vi "[RT] Finite Acq wSubset Reads.vi"() -> ()   [LabVIEW 2015]
doc: "A finite acquisition allocates exactly enough memory to hold all of the requested samples per channel. The rwfm_Read(poly).vi has a control named \"Samps Read per Chan\" that you can use to specify the block size returned by each Read call. In effect you can read a large finite acquisition in multiple small subsets."
uses:
  <vilib>/rvi/interface/nirviOpenFPGA/nirviOpenFPGA.xnode
  <vilib>/rvi/interface/nirviCloseFPGA/nirviCloseFPGA.xnode
  <vilib>/NI/cRIO Wfm/cRIO Wfm.lvlib
  <vilib>/NI/cRIO Wfm/AcqRead(Wfm).vi
  C/Program Files (x86)/National Instruments/LabVIEW 2015/ProjectTemplates/Source/cRIOWfm/FPGA Bitfiles/DeltaSigMain_9074.lvbitx
  C:/Program Files (x86)/National Instruments/LabVIEW 2015/ProjectTemplates/Source/cRIOWfm/FPGA/[FPGA] DeltaSig Main.vi
  C/Program Files (x86)/National Instruments/LabVIEW 2015/ProjectTemplates/Source/cRIOWfm/FPGA Bitfiles/SARAcqMain_9074.lvbitx
  C:/Program Files (x86)/National Instruments/LabVIEW 2015/ProjectTemplates/Source/cRIOWfm/FPGA/[FPGA] SAR Acq Main.vi
  <vilib>/NI/cRIO Wfm/DynamicFPGAref.ctl
  <vilib>/FPGAPlugInAG/Dynamic/niLvFpga_Close_Dynamic.vi
  <vilib>/NI/cRIO Wfm/ChannelConfig.ctl
panel:
  in  "Sample Rate":u32=51200
  in  "Channel Info":T1=[{"Channel Name"="Mod1/ai0", "Sensitivity mV_EU"=1000.0, "EU"="V", "dB Ref EU"=1.0}, {"Channel Name"="Mod1/ai1", "Sensitivity mV_EU"=1000.0, "EU"="V", "dB Ref EU"=1.0}, {"Channel Name"="Mod1/ai2", "Sensitivity mV_EU"=1000.0, "EU"="V", "dB Ref EU"=1.0}, {"Channel Name"="Mod1/ai3", "Sensitivity mV_EU"=1000.0, "EU"="V", "dB Ref EU"=1.0}] caption="Channel Name      Scale [mV/EU]        EU           dB Ref [EU]" {"dB Ref EU" format="%#.2p"; "Sensitivity mV_EU" format="%.2f"}
  out "Subsets Read":i32
  out "Buffer Backlog":dbl=nan caption="RT Buffer Backlog [%]"
  in  "Read Subsets":i32=5
  out "Waveform Graph":waveform(sgl)[](graph)
  in  "Samps per Chan":i32=102400 caption="Samples per Channel"
  # "Sampling Info"
  # "Channel Info"
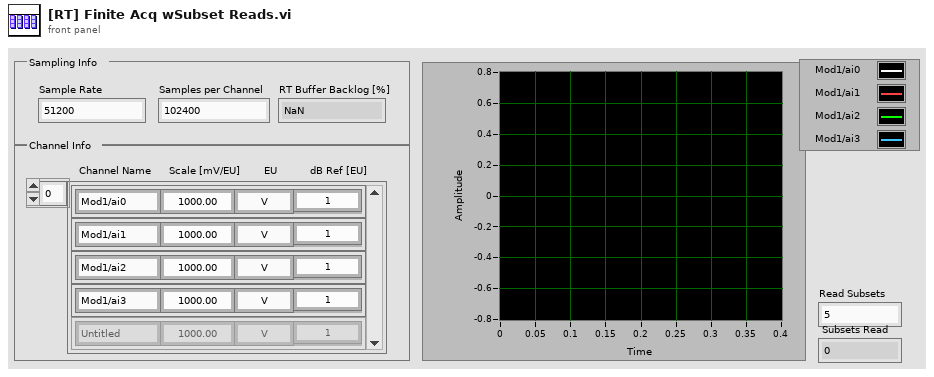
[diagram p1: front panel]
types:
  T1 = typedef "cRIO Wfm.lvlib/ChannelConfig.ctl" = cluster{"Channel Name":string, "Sensitivity mV_EU":dbl, "EU":string, "dB Ref EU":dbl}[]
  T2 = typedef "cRIO Wfm.lvlib/SamplingInfo.ctl" = cluster{"Number of Channels":i32, "Actual Samp Rate":dbl, "Chan Name Array":string[], "EU Chan Array":string[], "dB Ref Chan Array":dbl[]}
  T3 = typedef "cRIO Wfm.lvlib/DynamicFPGAref.ctl" = refnum<k20>
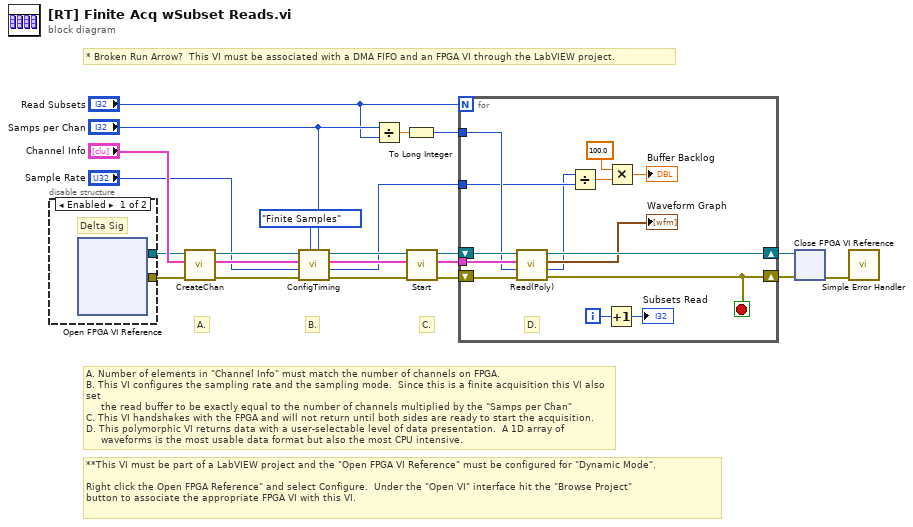
[diagram p0: block diagram]
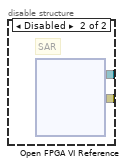
[diagram p2: hidden frame]
diagram:
  # "A. Number of elements in \"Channel Info\" must match the number of channels on FPGA.\nB. This VI configures the sampling rate and the sampling mode.  Since this is a finite acquisition this VI also set  \n     the read buffer to be exactly equal to the number of channels multiplied by the \"Samps per Chan\"\nC. This VI handshakes with the FPGA and will not return until both sides are ready to start the acquisition.\nD. This polymorphic VI returns data with a user-selectable level of data presentation.  A 1D array of     \n     waveforms is the most usable data format but also the most CPU intensive."
  # "**This VI must be part of a LabVIEW project and the \"Open FPGA VI Reference\" must be configured for \"Dynamic Mode\".\n\nRight click the Open FPGA Reference\" and select Configure.  Under the \"Open VI\" interface hit the \"Browse Project\" \nbutton to associate the appropriate FPGA VI with this VI."
  # "* Broken Run Arrow?  This VI must be associated with a DMA FIFO and an FPGA VI through the LabVIEW project."
  # "A."
  # "C."
  # "B."
  n1 = disable-structure shown="Enabled" {
    disable-tunnel: [w24 w26] -> w2
    disable-tunnel: [w23 w25] -> w1
    frame Enabled {
      # "Delta Sig"
      n2 = xnode "Open FPGA VI Reference"() -> ("FPGA VI Reference Out"=w24:refnum<k20>, "error out"=w23:errorcluster)  [unwired: 2 in]
    }
    frame Disabled {
      # "SAR"
      n3 = xnode "Open FPGA VI Reference"() -> ("FPGA VI Reference Out"=w26:refnum<k20>, "error out"=w25:errorcluster)  [unwired: 2 in]
    }
  }
  n4 = call <vilib>:"CreateChan.vi"("error in"=w1, "Channel Info"="Channel Info", "Dynamic FPGA Ref"=w2) -> ("error out"=w19:errorcluster, "Sampling Info"=w18:T2, "Dynamic FPGA Ref Out"=w20:T3)  [unwired: 1 in, 5 out]
  n5 = call <vilib>:"ConfigTiming.vi"("Samples per Channel"="Samps per Chan", "Sample Mode"=enum16{"Finite Samples", "Continuous Samples"}."Finite Samples", "error in"=w19, "Sample Rate"="Sample Rate", "Sampling Info In"=w18, "Dynamic FPGA Ref"=w20) -> ("error out"=w12:errorcluster, "Buffer Size [Total Samples]"=w5:u32, "Sampling Info Out"=w13:T2, "Dynamic FPGA Ref Out"=w14:T3)  [unwired: 2 in]
  n6 = Divide(x="Samps per Chan", y="Read Subsets") -> (x/y=w7:dbl)
  n7 = To Long Integer(number=w7) -> (32bit integer=w6:i32)
  n8 = call <vilib>:"Start.vi"("error in"=w12, "Sampling Info In"=w13, "Dynamic FPGA Ref"=w14) -> ("error out"=w16:errorcluster, "Sampling Info Out"=w17:T2, "Dynamic FPGA Ref Out"=w15:T3)  [unwired: 6 out]
  n9 = for {
    N: "Read Subsets" -> [_]
    tunnel: w17 -> [w40]
    shift-right: [w27] -> w10
    shift-left: w16 -> [w39]
    tunnel: w6 -> [w35]
    tunnel: w5 -> [w34]
    shift-right: [w37] -> w11
    shift-left: w15 -> [w38]
    i -> [w32]
    stop <- w27 stop-if-true
    # "D."
    n10 = call-poly <vilib>:"Read(Poly).vi"("error in"=w39, "Samps Read per Chan"=w35, "Sampling Info"=w40, "Dynamic FPGA Ref"=w38) -> ("error out"=w27:errorcluster, "Samples Remaining"=w33:u32, "Wfm Data"=→"Waveform Graph":waveform(sgl)[], "Dynamic FPGA Ref Out"=w37:T3)  [unwired: 2 in, 2 out]
    n11 = Divide(x=w33, y=w34) -> (x/y=w30:dbl)
    n12 = Increment(x=w32) -> (x+1=→"Subsets Read":i32)
    n13 = Multiply(x=100.0, y=w30) -> (x*y=→"Buffer Backlog":dbl)
  }
  n14 = xnode "Close FPGA VI Reference"("FPGA VI Reference In"=w11, "error in"=w10) -> ("error out"=w21:errorcluster)
  n15 = call <vilib>:"Simple Error Handler.vi"("error in (no error)"=w21) -> ()  [unwired: 1 in, 8 out]
